vi "Z900_navX_Get_SystemInformation_BoardInformation.vi"(8 "error in (no error)":errorcluster, 11 "navX Device":T4={"Interface"={"Protocol"=enum."SERIAL", "Update Rate (4Hz-60Hz)"=4, "navX Open TypeDef"=variant}, "Notify Packet"=refnum, "Loop VI Refnum"=refnum, "Ready to Close Occurrence Refnum"=refnum} {"Interface"."Update Rate (4Hz-60Hz)" min=4 max=60 step=1}) -> (0 "error out":errorcluster, 1 "Connected":bool, 2 "Board Information":T3 {"Board"."Hardware Revision" items=["navX-MXP"=33, "navX-Micro"=40]; "Omnimount Config" items=["DEFAULT", "X_UP", "X_DOWN", "Y_UP", "Y_DOWN", "Z_UP", "Z_DOWN"]}, 3 "navX Device":T4={"Interface"={"Protocol"=enum."SERIAL", "Update Rate (4Hz-60Hz)"=4, "navX Open TypeDef"=variant}, "Notify Packet"=refnum, "Loop VI Refnum"=refnum, "Ready to Close Occurrence Refnum"=refnum} {"Interface"."Update Rate (4Hz-60Hz)" min=4 max=60 step=1})   [LabVIEW 2015, in "navX Library v2.lvlib"]
doc: "This navX VI will return the current Board Information.\nWho Am I\nHardware Revision\nFirmware Major and Minor\nCapability\nOmnimount Config"
uses:
  navX Library v2.lvlib
  TypeDefs/Z900_navX_DeviceTypeDef.ctl
  TypeDefs/Z900_navX_ProtocolTypeDef.ctl
  TypeDefs/Z900_navX_NotifyPacketTypeDef.ctl
  TypeDefs/Z900_navX_ActionTypeDef.ctl
  TypeDefs/Flags/Z900_navX_Flags_HardwareRevTypeDef.ctl
  TypeDefs/Flags/Z900_navX_Flags_OmnimountConfigTypeDef.ctl
  TypeDefs/Z900_navX_DeviceRegisters.ctl
  TypeDefs/Flags/Z900_navX_Flags_CapabilityTypeDef.ctl
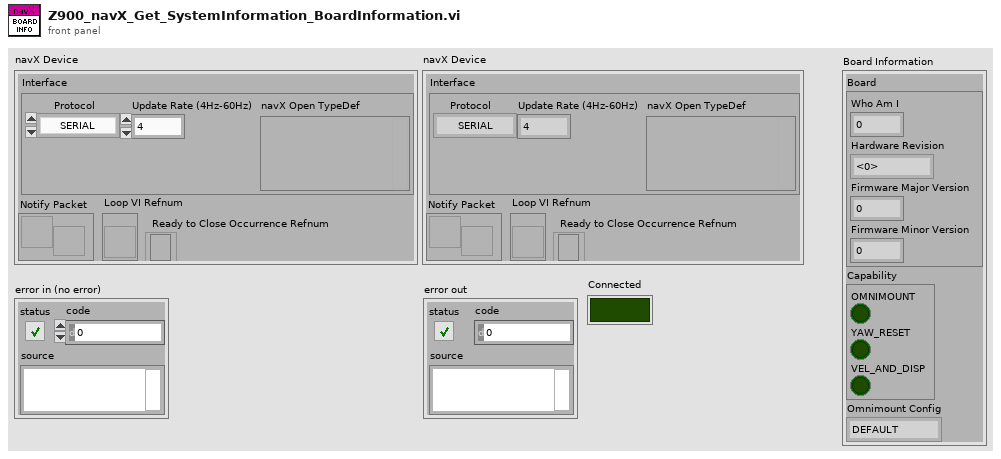
[diagram p1: front panel]
types:
  T1 = typedef "navX Library v2.lvlib/Z900_navX_Flags_HardwareRevTypeDef.ctl" = u8
  T2 = typedef "navX Library v2.lvlib/Z900_navX_Flags_OmnimountConfigTypeDef.ctl" = u8
  T3 = cluster{"Board":cluster{"Who Am I":u8, "Hardware Revision":T1, "Firmware Major Version":u8, "Firmware Minor Version":u8}, "Capability":cluster{"OMNIMOUNT":bool, "YAW_RESET":bool, "VEL_AND_DISP":bool}, "Omnimount Config":T2}
  T4 = typedef "navX Library v2.lvlib/Z900_navX_DeviceTypeDef.ctl" = cluster{"Interface":cluster{"Protocol":T5, "Update Rate (4Hz-60Hz)":u8, "navX Open TypeDef":variant}, "Notify Packet":refnum<notifier>, "Loop VI Refnum":refnum<vi>, "Ready to Close Occurrence Refnum":refnum<k4>}
  T5 = typedef "navX Library v2.lvlib/Z900_navX_ProtocolTypeDef.ctl" = enum16{"SERIAL", "I2C", "SPI"}
  T6 = cluster{"Who Am I":u8, "Hardware Revision":T1, "Firmware Major Version":u8, "Firmware Minor Version":u8}
  T7 = cluster{"OMNIMOUNT":bool, "YAW_RESET":bool, "VEL_AND_DISP":bool}
  T8 = typedef "navX Library v2.lvlib/Z900_navX_DeviceRegisters.ctl" = u8
  T9 = typedef "navX Library v2.lvlib/Z900_navX_Flags_CapabilityTypeDef.ctl" = u16
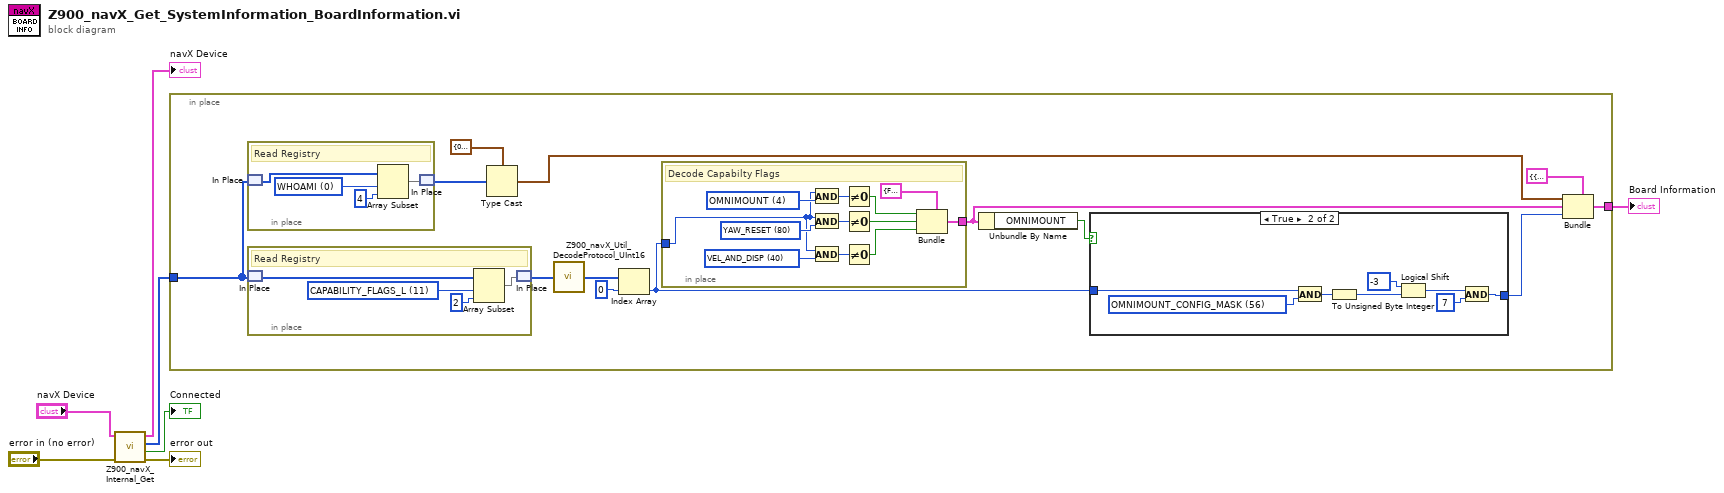
[diagram p0: block diagram]
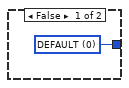
[diagram p2: hidden frame]
diagram:
  n1 = call "Z900_navX_Internal_Get.vi"("error in (no error)"="error in (no error)", "navX Device"="navX Device") -> ("error out"=→"error out":errorcluster, "Connected"=→"Connected":bool, "Registry"=w3:u8[], "navX Device"=→"navX Device":T4)  [unwired: 6 in]
  n2 = in-place {
    in-place-border: w3 -> [w16]
    in-place-border: [w10] -> w2
    n3 = in-place {
      w23 = T8 0 items=["WHOAMI"=0, "HW_REV"=1, "FW_VER_MAJOR"=2, "FW_VER_MINOR"=3, "UPDATE_RATE_HZ"=4, "ACCEL_FSR_G"=5, "GYRO_FSR_DPS"=6, "OP_STATUS"=8, "CAL_STATUS"=9, "SELFTEST_STATUS"=10, "CAPABILITY_FLAGS_L"=11, "CAPABILITY_FLAGS_H"=12, "SENSOR_STATUS"=16, "TIMESTAMP"=18, "YAW"=22, "ROLL"=24, "PITCH"=26, "HEADING"=28, "FUSED_HEADING"=30, "ALTITUDE_I"=32, "ALTITUDE_D"=34, "LINERA_ACC_X"=36, "LINERA_ACC_Y"=38, "LINERA_ACC_Z"=40, "QUAT_W"=42, "QUAT_X"=44, "QUAT_Y"=46, "QUAT_Z"=48, "MPU_TEMP_C"=50, "GYRO_X"=52, "GYRO_Y"=54, "GYRO_Z"=56, "ACC_X"=58, "ACC_Y"=60, "ACC_Z"=62, "MAG_X"=64, "MAG_Y"=66, "MAG_Z"=68, "PRESSURE_I"=70, "PRESSURE_D"=72, "PRESSURE_TEMP"=74, "YAW_OFFSET"=76, "QUAT_OFFSET_W"=78, "QUAT_OFFSET_X"=80, "QUAT_OFFSET_Y"=82, "QUAT_OFFSET_Z"=84, "INTEGRATION_CONTROL"=86, "VELOCITY_X"=88, "VELOCITY_Y"=92, "VELOCITY_Z"=96, "DISPLACMENT_X"=100, "DISPLACMENT_Y"=104, "DISPLACEMENT_Z"=108] ("Device Register")
      # "Read Registry"
      n4 = in-place-match #1(w16) -> (w21:u8[])
      n5 = Array Subset(array=w21, index=w23, length=4) -> (w22:u8[])
      n6 = in-place-match #1(w22) -> (w15:u8[])
    }
    n7 = in-place {
      w48 = T8 11 items=["WHOAMI"=0, "HW_REV"=1, "FW_VER_MAJOR"=2, "FW_VER_MINOR"=3, "UPDATE_RATE_HZ"=4, "ACCEL_FSR_G"=5, "GYRO_FSR_DPS"=6, "OP_STATUS"=8, "CAL_STATUS"=9, "SELFTEST_STATUS"=10, "CAPABILITY_FLAGS_L"=11, "CAPABILITY_FLAGS_H"=12, "SENSOR_STATUS"=16, "TIMESTAMP"=18, "YAW"=22, "ROLL"=24, "PITCH"=26, "HEADING"=28, "FUSED_HEADING"=30, "ALTITUDE_I"=32, "ALTITUDE_D"=34, "LINERA_ACC_X"=36, "LINERA_ACC_Y"=38, "LINERA_ACC_Z"=40, "QUAT_W"=42, "QUAT_X"=44, "QUAT_Y"=46, "QUAT_Z"=48, "MPU_TEMP_C"=50, "GYRO_X"=52, "GYRO_Y"=54, "GYRO_Z"=56, "ACC_X"=58, "ACC_Y"=60, "ACC_Z"=62, "MAG_X"=64, "MAG_Y"=66, "MAG_Z"=68, "PRESSURE_I"=70, "PRESSURE_D"=72, "PRESSURE_TEMP"=74, "YAW_OFFSET"=76, "QUAT_OFFSET_W"=78, "QUAT_OFFSET_X"=80, "QUAT_OFFSET_Y"=82, "QUAT_OFFSET_Z"=84, "INTEGRATION_CONTROL"=86, "VELOCITY_X"=88, "VELOCITY_Y"=92, "VELOCITY_Z"=96, "DISPLACMENT_X"=100, "DISPLACMENT_Y"=104, "DISPLACEMENT_Z"=108] ("Device Register")
      # "Read Registry"
      n8 = in-place-match #2(w16) -> (w46:u8[])
      n9 = Array Subset(array=w46, index=w48, length=2) -> (w47:u8[])
      n10 = in-place-match #2(w47) -> (w20:u8[])
    }
    n11 = Type Cast(type=T6 {"Who Am I"=0, "Hardware Revision"=33, "Firmware Major Version"=0, "Firmware Minor Version"=0}, x=w15) -> (*(type *) &x=w11:T6)
    n12 = call "Z900_navX_Util_DecodeProtocol_UInt16.vi"("Little Endian"=w20) -> ("UInt16"=w19:u16[])
    n13 = Index Array(array=w19, index=0) -> (element=w18:u16)
    n14 = in-place {
      in-place-border: w18 -> [w36]
      in-place-border: [w34] -> w12
      w39 = T9 40 items=["OMNIMOUNT"=4, "OMNIMOUNT_CONFIG_MASK"=38, "VEL_AND_DISP"=40, "YAW_RESET"=80] ("Capability Flag")
      w40 = T9 80 items=["OMNIMOUNT"=4, "OMNIMOUNT_CONFIG_MASK"=38, "VEL_AND_DISP"=40, "YAW_RESET"=80] ("Capability Flag")
      w45 = T9 4 items=["OMNIMOUNT"=4, "OMNIMOUNT_CONFIG_MASK"=38, "VEL_AND_DISP"=40, "YAW_RESET"=80] ("Capability Flag")
      # "Decode Capabilty Flags"
      n15 = And(x=w36, y=w45) -> (x .and. y?=w44:T9)
      n16 = And(x=w36, y=w40) -> (x .and. y?=w41:T9)
      n17 = And(x=w36, y=w39) -> (x .and. y?=w38:T9)
      n18 = Not Equal To 0?(x=w44) -> (x != 0?=w42:bool)
      n19 = Not Equal To 0?(x=w41) -> (x != 0?=w37:bool)
      n20 = Not Equal To 0?(x=w38) -> (x != 0?=w35:bool)
      n21 = Bundle(cluster=T7 {"OMNIMOUNT"=FALSE, "YAW_RESET"=FALSE, "VEL_AND_DISP"=FALSE}, "OMNIMOUNT"=w42, "YAW_RESET"=w37, "VEL_AND_DISP"=w35) -> (w34:T7)
    }
    n22 = Unbundle By Name(w12) -> ("OMNIMOUNT"=w17:bool)
    n23 = case shown="True" w17 {
      tunnel: [w25 w27] -> w8
      tunnel: w18 -> [_ w33]
      frame False {
        w25 = u8 0 items=["DEFAULT", "X_UP", "X_DOWN", "Y_UP", "Y_DOWN", "Z_UP", "Z_DOWN"] ("OMNIMOUNT_CONFIG")
      }
      frame True {
        w32 = T9 56 items=["OMNIMOUNT"=4, "OMNIMOUNT_CONFIG_MASK"=56, "VEL_AND_DISP"=64, "YAW_RESET"=128] ("Capability Flag")
        n24 = And(x=w33, y=w32) -> (x .and. y?=w31:T9)
        n25 = To Unsigned Byte Integer(number=w31) -> (unsigned 8bit integer=w26:u8)
        n26 = Logical Shift(y=-3, x=w26) -> (x << y=w29:u8)
        n27 = And(x=w29, y=7) -> (x .and. y?=w27:i32)
      }
    }
    n28 = Bundle(cluster=T3 {"Board"={"Who Am I"=0, "Hardware Revision"=33, "Firmware Major Version"=0, "Firmware Minor Version"=0}, "Capability"={"OMNIMOUNT"=FALSE, "YAW_RESET"=FALSE, "VEL_AND_DISP"=FALSE}, "Omnimount Config"=0}, "Board"=w11, "Capability"=w12, "Omnimount Config"=w8) -> (w10:T3)
  }
  "Board Information" <- w2
